vi "List.vi"(8 "error in (no error)":errorcluster, 11 "CloneRegRef":refnum<data-value>) -> (0 "error out":errorcluster, 1 "First? (all)":bool[](array[boolean]), 2 "Found?":bool, 3 "CloneRegRef":refnum<data-value>, 4 "Module IDs":i32[](array[numeric]), 5 "Instance Names":string[](array[string]))   [LabVIEW 2014, in "ModuleAdmin.lvlib" / "CloneRegistration.lvclass"]
uses:
  CloneRegistration.lvclass
  CloneRegistration.lvclass/CloneRegistration.ctl
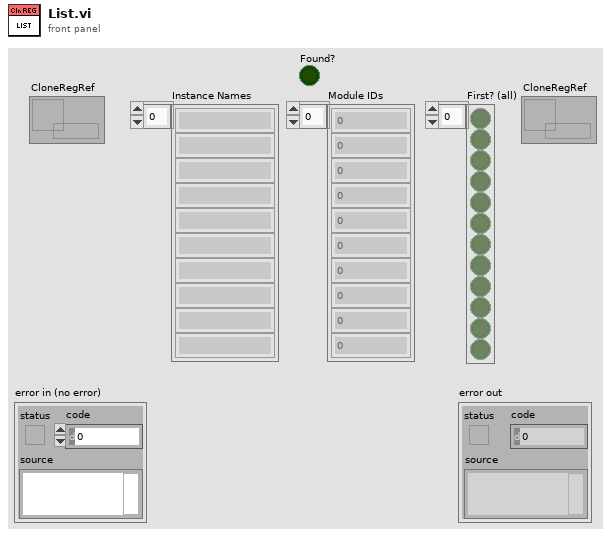
[diagram p1: front panel]
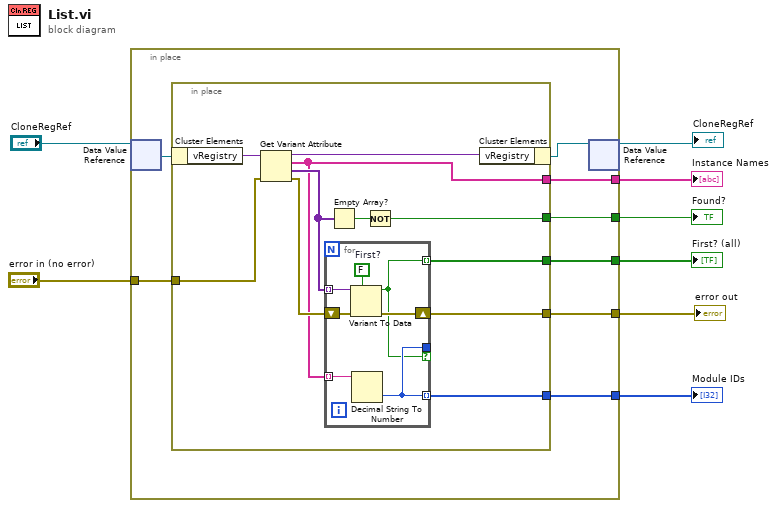
[diagram p0: block diagram]
diagram:
  n1 = in-place {
    in-place-border: [w16] -> w8
    in-place-border: [w15] -> w7
    in-place-border: "error in (no error)" -> [w14]
    in-place-border: [w13] -> w5
    in-place-border: [w12] -> w4
    in-place-border: [w11] -> w3
    n2 = in-place-dvr #1("CloneRegRef") -> (w10:refnum<class "CloneRegistration.lvclass">)  [unwired: 1 out]
    n3 = in-place {
      in-place-border: [w22] -> w16
      in-place-border: [w21] -> w15
      in-place-border: w14 -> [w20]
      in-place-border: [w19] -> w13
      in-place-border: [w18] -> w12
      in-place-border: [w17] -> w11
      n4 = in-place-cluster #2(w10) -> ("vRegistry"=w27:variant)
      n5 = Get Variant Attribute(Variant=w27, error in=w20) -> (duplicate Variant=w26:variant, names=w19:string[], values=w23:variant[], error out=w25:errorcluster)  [unwired: 2 in]
      n6 = for {
        tunnel: w19 -> [w34] mode=indexing
        tunnel: [w29] -> w18 mode=indexing
        tunnel: w23 -> [w33] mode=indexing
        shift-right: [w30] -> w21
        shift-left: w25 -> [w31]
        tunnel: [w28] -> w17 mode=indexing
        tunnel: [w29] -> _ if=w28
        w32 = FALSE  # First?
        n7 = Variant To Data(error in=w31, type=w32, Variant=w33) -> (data=w28:bool, error out=w30:errorcluster)
        n8 = Decimal String To Number(string=w34) -> (number=w29:i32)  [unwired: 2 in, 1 out]
      }
      n9 = Empty Array?(array=w23) -> (empty?=w24:bool)
      n10 = Not(x=w24) -> (.not. x?=w22:bool)
      n11 = in-place-cluster #2("vRegistry"=w26) -> (w9:refnum<class "CloneRegistration.lvclass">)
    }
    n12 = in-place-dvr #1(w9) -> (→"CloneRegRef":refnum<data-value>)  [unwired: 1 out]
  }
  "error out" <- w7
  "Found?" <- w8
  "Instance Names" <- w5
  "Module IDs" <- w4
  "First? (all)" <- w3
